vi "GetSfxDLData_Addon.vi"(6 "Resp Timeout (ms)":i32 min=0, 7 "Active Dut":T1, 8 "Error In":errorcluster, 11 "FPGA Reference":refnum<k20>) -> (0 "Error Out":errorcluster, 2 "RxTestmode OK":bool, 3 "test_mode_resp":string)   [LabVIEW 2018]
uses:
  Resources_Test/UART/ControlTestSlot.ctl
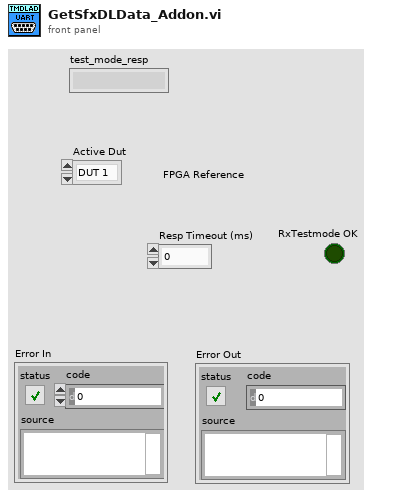
[diagram p1: front panel]
types:
  T1 = typedef "ControlTestSlot.ctl" = enum16{"DUT 1", "DUT 2"}
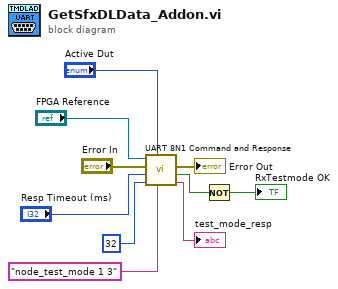
[diagram p0: block diagram]
diagram:
  n1 = call "UART 8N1 Command and Response.vi"("Text to Send"="node_test_mode 1 3", "Active Dut"="Active Dut", "Response Size (char)"=u32 32, "Response Timeout (ms)"="Resp Timeout (ms)", "Error In"="Error In", "FPGA VI Reference In"="FPGA Reference") -> ("Received Text"=→"test_mode_resp":string, "Timeout Flag"=w9:bool, "Error Out"=→"Error Out":errorcluster)  [unwired: 1 in, 2 out]
  n2 = Not(x=w9) -> (.not. x?=→"RxTestmode OK":bool)
